vi "get channels.vi"(11 "Logic Sequencer configuration in":refnum<class "Logic Sequencer configuration.lvclass">) -> (2 "channels":refnum<class "TBM channel.lvclass">[](array[class]), 3 "Logic Sequencer configuration out":refnum<class "Logic Sequencer configuration.lvclass">)   [LabVIEW 2013, in "Logic Sequencer configuration.lvclass"]
uses:
  Logic Sequencer configuration.lvclass
  <vilib>/NI/Tag Bus Module Framework/channel/TBM channel.lvclass
  Logic Sequencer configuration.lvclass/Logic Sequencer configuration.ctl
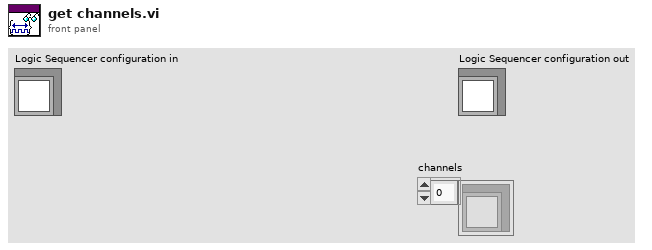
[diagram p1: front panel]
types:
  T1 = typedef "Logic Sequencer configuration.lvclass/processing channels.ctl" = cluster{"parameter":refnum<class "TBM channel.lvclass">, "result":refnum<class "TBM channel.lvclass">}
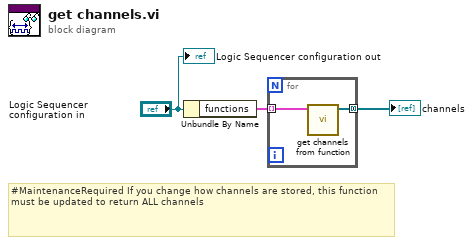
[diagram p0: block diagram]
diagram:
  # "#MaintenanceRequired If you change how channels are stored, this function must be updated to return ALL channels"
  n1 = Unbundle By Name("Logic Sequencer configuration in") -> ("functions"=w2:T1[])
  n2 = for {
    tunnel: w2 -> [w4] mode=indexing
    tunnel: [w5] -> w1 mode=concatenating
    n3 = call "get channels from function.vi"("processing function"=w4) -> ("channels"=w5:refnum<class "TBM channel.lvclass">[])  [unwired: 10 in]
  }
  "channels" <- w1
  "Logic Sequencer configuration out" <- "Logic Sequencer configuration in"
